vi "test_20SimModel.vi"() -> ()   [LabVIEW 2011]
uses:
  <vilib>/Platform/TimedLoop/XDataNode/timing_clust.ctl
  <vilib>/Platform/TimedLoop/XDataNode/nitl_modes.ctl
  <vilib>/Platform/TimedLoop/XDataNode/wakeup.ctl
  20SimModelRunStates.ctl
  <vilib>/Platform/TimedLoop/XDataNode/XDataNode.xnode
  <vilib>/Platform/TimedLoop/XDataNode/XDNodeRunTimeDep.lvlib
panel:
  in  "Input 1":dbl(slide) scale=-10.0..10.0
  in  "Set finish time {s}":dbl=-1.0
  in  "Set plot range {s}":dbl=10.0
  out "stepsize":dbl
  out "finishtime":dbl
  out "starttime":dbl
  out "DLL returnvalue":i32
  out "time":dbl
  out "Model outputs":T1(graph)
  in  "Stop the model":bool
  # "Example Labview model showing how to incorporate a 20-sim model in a Labview VI"
  # "Model settings"
  # "Settings retrieved from 20-sim model"
  # "-1 = infinite"
  # "Model inputs"
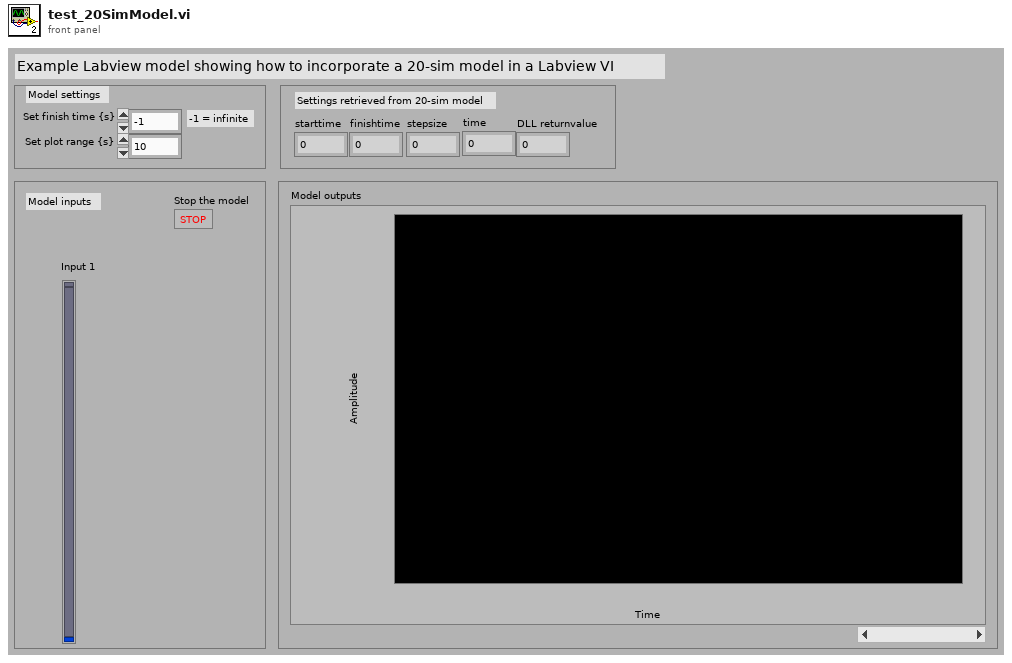
[diagram p1: front panel]
types:
  T1 = cluster{"outarr[0]":dbl, "outarr[1]":dbl, "outarr[2]":dbl, "outarr[3]":dbl, "outarr[4]":dbl, "outarr[5]":dbl, "outarr[6]":dbl, "outarr[7]":dbl, "outarr[8]":dbl}
  T2 = typedef "XDNodeRunTimeDep.lvlib/timing_clust.ctl" = cluster{"Expected End [f-1]":u64, "Actual End [f-1]":u64, "Finished Late? [f-1]":bool, "Expected End [i-1]":u64, "Actual End [i-1]":u64, "Finished Late? [i-1]":bool, "Expected Start [i]":u64, "Actual Start [i]":u64, "Expected Start [f]":u64, "Actual Start [f]":u64, "Source Name":string, "Structure Name":string, "Period":i64, "Deadline":i64, "Offset":i64, "Start":i64, "Priority":i32, "Timeout":i32, "Mode":T3, "Wakeup Reason":T4, "Error":errorcluster, "Source Type":string, "Secondary Source Type":string, "Global End Time":u64, "Global Start Time":u64, "Frame Duration":u64, "Iteration Duration":u64, "Assigned CPU":i32, "I/O Scan Engine Mode":u32}
  T3 = typedef "XDNodeRunTimeDep.lvlib/nitl_modes.ctl" = enum32{"No Change", "Process missed periods, maintain original phase", "Discard missed periods, maintain original phase", "Process missed periods, ignore original phase", "Discard missed periods, ignore original phase"}
  T4 = typedef "XDNodeRunTimeDep.lvlib/wakeup.ctl" = enum32{"Normal", "Aborted", "Asynchronous wakeup", "Timing source error", "Timed loop error", "Timeout"}
  T5 = cluster{"OutputsArray[0]":dbl, "OutputsArray[1]":dbl, "OutputsArray[2]":dbl, "OutputsArray[3]":dbl, "OutputsArray[4]":dbl, "OutputsArray[5]":dbl, "OutputsArray[6]":dbl, "OutputsArray[7]":dbl, "OutputsArray[8]":dbl}
  T6 = cluster{"OutputsArray[0]":dbl, "OutputsArray[1]":dbl, "OutputsArray[2]":dbl, "OutputsArray[3]":dbl, "OutputsArray[4]":dbl, "OutputsArray[5]":dbl, "OutputsArray[6]":dbl, "OutputsArray[7]":dbl, "OutputsArray[8]":dbl}[]
  T7 = typedef "20SimModelRunStates.ctl" = enum16{"Init", "Run", "Terminate", "Error"}
  T8 = cluster{"[0]":dbl, "[1]":dbl, "[2]":dbl, "[3]":dbl, "[4]":dbl, "[5]":dbl, "[6]":dbl, "[7]":dbl, "[8]":dbl}
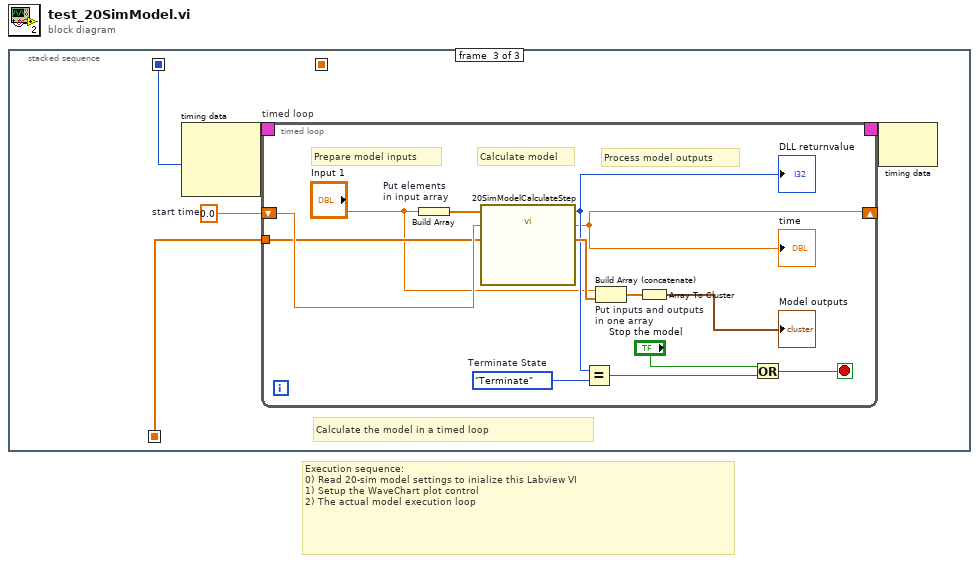
[diagram p0: block diagram]
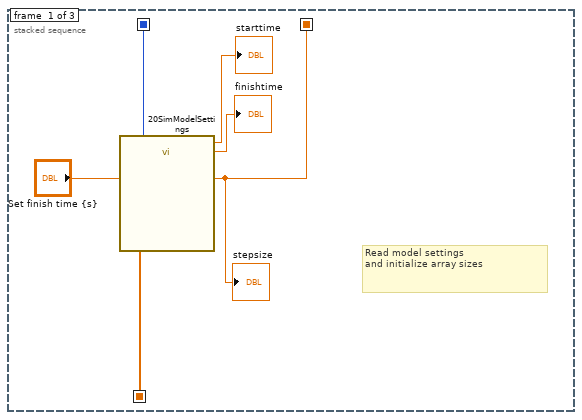
[diagram p2: hidden frame]
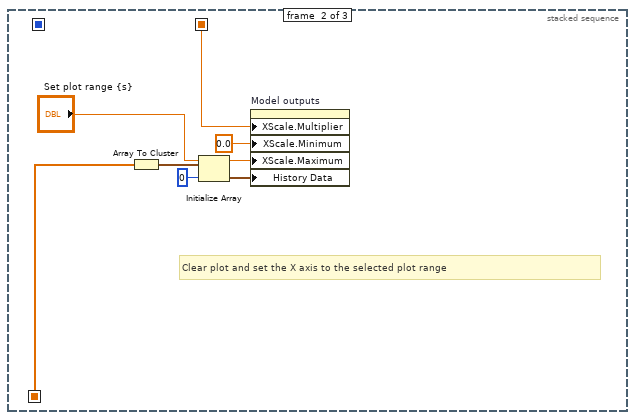
[diagram p3: hidden frame]
diagram:
  # "Execution sequence:\n0) Read 20-sim model settings to inialize this Labview VI\n1) Setup the WaveChart plot control\n2) The actual model execution loop"
  n1 = stacked-sequence {
    seq-local: [w3 _ _] -> [_ w7 w16]
    seq-local: [w2 _ _] -> [_ _ w15]
    seq-local: [w1 _ _] -> [_ w8 _]
    frame #0 {
      # "Read model settings\nand initialize array sizes"
      n2 = call "20SimModelSettings.vi"("Set finish time"="Set finish time {s}") -> ("period_ms"=w2:i32, "OutputsArray"=w3:dbl[], "finishtime"=→"finishtime":dbl, "starttime"=→"starttime":dbl, "stepsize"=w1:dbl)  [unwired: 3 in, 3 out]
      "stepsize" <- w1
    }
    frame #1 {
      # "Clear plot and set the X axis to the selected plot range"
      n3 = Array To Cluster(array=w7) -> (cluster=w9:T5)
      n4 = Initialize Array(w9, 0) -> (w13:T6)
      n5 = property on="Model outputs" class="WFChart (strict)"("XScale.Multiplier"=w8, "XScale.Minimum"=0.0 ("X Scale.Range:Minimum"), "XScale.Maximum"="Set plot range {s}", "History Data"=w13) -> ()  [unwired: 2 in, 2 out]
    }
    frame #2 {
      w14 = 0.0  # start time
      # "Calculate the model in a timed loop"
      n6 = node-c288(w15) -> (w18:T2)  [unwired: 2 out]
      n7 = timed-loop "timed loop" {
        timing: w18 -> [_]
        timing-out: [_] -> w17
        shift-right: [w25] -> _
        shift-left: w14 -> [w24]
        tunnel: w16 -> [w22]
        stop <- w23 stop-if-true
        w31 = 20SimModelRunStates."Terminate"  # Terminate State
        # "Process model outputs"
        # "Calculate model"
        # "Prepare model inputs"
        n8 = Build Array "Put elements\nin input array"("Input 1") -> (w28:dbl[])
        n9 = call "20SimModelCalculateStep.vi"("OutputArrayInitial"=w22, "time in"=w24, "InputArray"=w28) -> ("OutputArray"=w30:dbl[], "time out"=w25:dbl, "ReturnValue"=w27:i32)  [unwired: 6 in]
        "time" <- w25
        "DLL returnvalue" <- w27
        n10 = Equal?(x=w27, y=w31) -> (x = y?=w20:bool)
        n11 = Build Array (concatenate) "Put inputs and outputs in one array"("Input 1", w30) -> (w29:dbl[])
        n12 = Array To Cluster(array=w29) -> (cluster=→"Model outputs":T8)
        n13 = Or(x="Stop the model", y=w20) -> (x .or. y?=w23:bool)
      }
      n14 = node-c288(w17) -> ()  [unwired: 1 out]
    }
  }
